vi "BRig_RT__Case_Exp__recordAnalogInput__PortA__fifo__1value.vi"(2 "input_iOccurence":u16, 3 "resetOccurrence":bool, 4 "input_dataCurrent":u16[](array[numeric]), 6 "input_iState_start":T1, 7 "rt fifo":refnum<k33>, 8 "input_iState_end":T1, 9 "input_fifo_error":errorcluster, 10 "input_AI1":u16, 12 "input_AI0":u16) -> (11 "output_fifo_error":errorcluster, 13 "rt fifo out":refnum<k33>, 16 "output_iOccurrence":u16)   [LabVIEW 2014]
uses:
  myRIO_BRig_RT__Case_Exp_stateList.ctl
panel:
  out "anyTimeout":bool
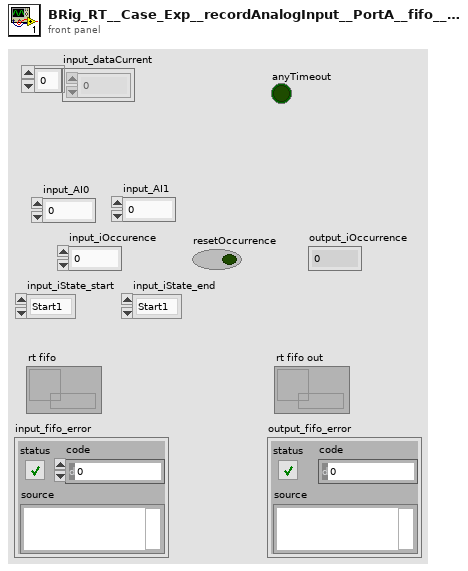
[diagram p1: front panel]
types:
  T1 = typedef "myRIO_BRig_RT__Case_Exp_stateList.ctl" = enum16{"Start1", "Start2", "Start3", "saveSettings1", "saveSettings2", "saveSettings3", "saveSettings4", "saveSettings_LC_ENL_l1", "saveSettings_LC_ENL_l2", "saveSettings_LC_Cue_l1", "saveSettings_LC_Cue_l2", "saveSettings6_LC_l1_Other", "SaveSettings6_LC_l2_Other", "setSettings_Audio", "setSettings_Laser", "initBlock_pre", "initBlock", "initBlock2", "initBlock_post", "initTrial_pre", "initTrial", "initTrial2", "initTrial3", "initTrial4", "initTrial_LC_ENL1", "initTrial_LC_Cue1", "initTrial_LC_Cue1_2", "initTrial_LC_Sel", "initTrial_post", "ENL1_pre", "ENL1", "ENL1_post", "ENL1Penalty_pre", "ENL1Penalty", "ENL2_pre", "ENL2", "ENL2Penalty_pre", "ENL2Penalty", "Cue1_pre", "Cue1", "Cue1_post", "Cue1Penalty_pre", "Cue1Penalty", "Cue2_pre", "Cue2", "Cue2Penalty_pre", "Cue2Penalty", "Selection_pre", "Selection", "Select_post", "SelectReward_pre", "SelectReward", "SelectRewardPost_pre", "SelectRewardPost", "SelectWrong_pre", "SelectWrong", "SelectWrong_post", "SelectTimeout_pre", "SelectTimeout", "SelectTimeout_post", "endTrial_pre", "endTrial1", "endTrial2", "endTrial3", "endTrial_post", "endBlock_pre", "endBlock", "endBlock_post", "endExp", "commConnect", "commUpload_pre", "commUpload_dataBlock", "commUpload_dataCurrent", "commUpload_dataExp", "commUpload_dataLC", "commUpload_dataTrial", "commUpload_post", "saveData_pre", "saveData_dataBlock", "saveData_dataCurrent", "saveData_dataExp", "saveData_dataLC", "saveData_dataTrial", "saveData_post", "empty_endBlock1", "empty_endBlock2", "empty_endTrial1", "empty_endTrial2", "empty_endTrial3", "empty_endTrial4", "empty_endTrial5", "dummyState", "dummyState_endBlock", "FreeReward_pre", "FreeReward", "FreeRewardPost_pre", "FreeRewardPost"}
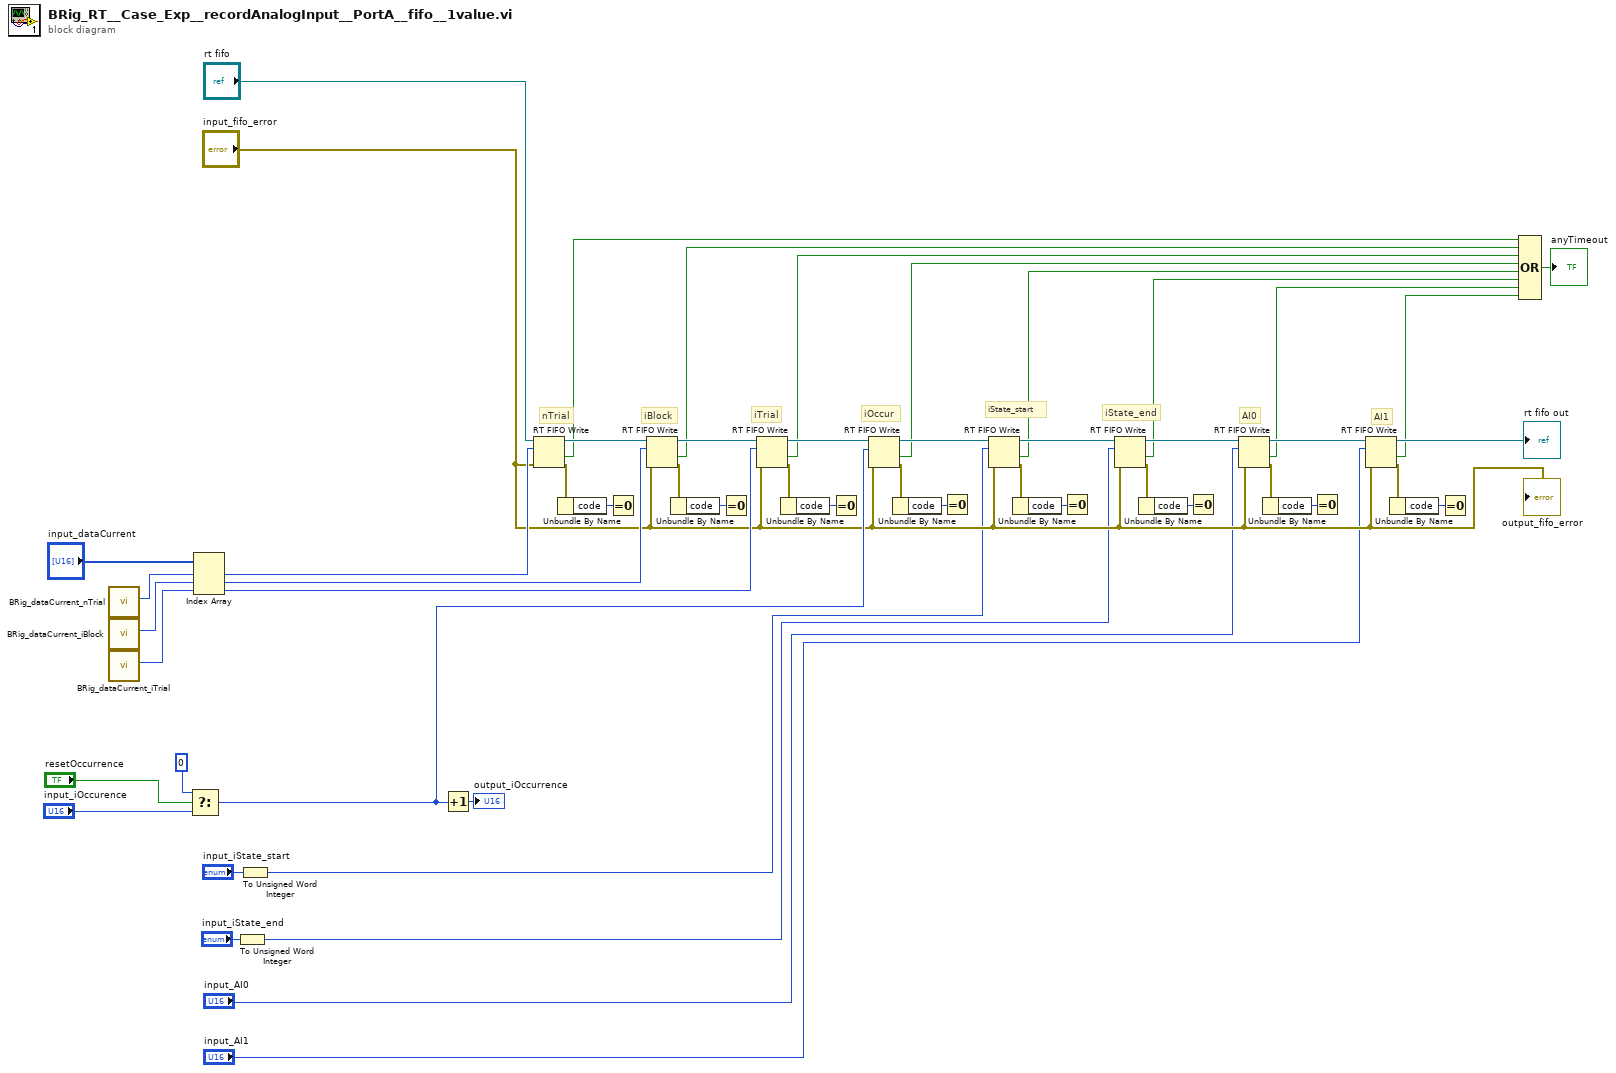
[diagram p0: block diagram]
diagram:
  # "AI1"
  # "AI0"
  # "iState_end"
  # "iState_start"
  # "iOccur"
  # "iTrial"
  # "iBlock"
  # "nTrial"
  n1 = call "BRig_dataCurrent_nTrial.vi"() -> ("output_nTrial"=w52:i32)  [unwired: 11 in]
  n2 = call "BRig_dataCurrent_iBlock.vi"() -> ("output_iBlock"=w51:i32)  [unwired: 11 in]
  n3 = call "BRig_dataCurrent_iTrial.vi"() -> ("output_iTrial"=w50:i32)  [unwired: 11 in]
  n4 = Select(t=u16 0, s="resetOccurrence", f="input_iOccurence") -> (s? t:f=w15:u16)
  n5 = Index Array(array="input_dataCurrent", index #1=w52, index #2=w51, index #3=w50) -> (element #1=w18:u16, element #2=w17:u16, element #3=w16:u16)
  n6 = To Unsigned Word Integer(number="input_iState_end") -> (unsigned 16bit integer=w12:u16)
  n7 = To Unsigned Word Integer(number="input_iState_start") -> (unsigned 16bit integer=w13:u16)
  n8 = Increment(x=w15) -> (x+1=→"output_iOccurrence":u16)
  n9 = RT FIFO Write(0:"rt fifo", 1:w18, 3:"input_fifo_error") -> (8:w36:refnum<k33>, 10:w4:bool, 11:w35:errorcluster)  [unwired: 2 in, 1 out]
  n10 = Unbundle By Name(w35) -> ("code"=w40:i32)
  n11 = Equal To 0?(x=w40) -> ()  [unwired: 1 out]
  n12 = RT FIFO Write(0:w36, 1:w17, 3:"input_fifo_error") -> (8:w32:refnum<k33>, 10:w5:bool, 11:w38:errorcluster)  [unwired: 2 in, 1 out]
  n13 = Unbundle By Name(w38) -> ("code"=w37:i32)
  n14 = Equal To 0?(x=w37) -> ()  [unwired: 1 out]
  n15 = RT FIFO Write(0:w32, 1:w16, 3:"input_fifo_error") -> (8:w29:refnum<k33>, 10:w6:bool, 11:w34:errorcluster)  [unwired: 2 in, 1 out]
  n16 = Unbundle By Name(w34) -> ("code"=w33:i32)
  n17 = Equal To 0?(x=w33) -> ()  [unwired: 1 out]
  n18 = RT FIFO Write(0:w29, 1:w15, 3:"input_fifo_error") -> (8:w26:refnum<k33>, 10:w7:bool, 11:w30:errorcluster)  [unwired: 2 in, 1 out]
  n19 = Unbundle By Name(w30) -> ("code"=w31:i32)
  n20 = Equal To 0?(x=w31) -> ()  [unwired: 1 out]
  n21 = RT FIFO Write(0:w26, 1:w13, 3:"input_fifo_error") -> (8:w23:refnum<k33>, 10:w8:bool, 11:w27:errorcluster)  [unwired: 2 in, 1 out]
  n22 = Unbundle By Name(w27) -> ("code"=w28:i32)
  n23 = Equal To 0?(x=w28) -> ()  [unwired: 1 out]
  n24 = RT FIFO Write(0:w23, 1:w12, 3:"input_fifo_error") -> (8:w20:refnum<k33>, 10:w9:bool, 11:w24:errorcluster)  [unwired: 2 in, 1 out]
  n25 = Unbundle By Name(w24) -> ("code"=w25:i32)
  n26 = Equal To 0?(x=w25) -> ()  [unwired: 1 out]
  n27 = RT FIFO Write(0:w20, 1:"input_AI0", 3:"input_fifo_error") -> (8:w19:refnum<k33>, 10:w10:bool, 11:w21:errorcluster)  [unwired: 2 in, 1 out]
  n28 = Unbundle By Name(w21) -> ("code"=w22:i32)
  n29 = Equal To 0?(x=w22) -> ()  [unwired: 1 out]
  n30 = RT FIFO Write(0:w19, 1:"input_AI1", 3:"input_fifo_error") -> (8:→"rt fifo out":refnum<k33>, 10:w11:bool, 11:w42:errorcluster)  [unwired: 2 in, 1 out]
  n31 = Unbundle By Name(w42) -> ("code"=w43:i32)
  n32 = Equal To 0?(x=w43) -> ()  [unwired: 1 out]
  n33 = Compound Arithmetic op=OR(w4, w5, w6, w7, w8, w9, w10, w11) -> (→"anyTimeout":bool)
  "output_fifo_error" <- "input_fifo_error"
